vi "ExSubSetPixelResTifFileHeader.vi"(3 "error in (no error)":errorcluster, 4 "Camera Handle":u32, 5 "File Handle":u32) -> (0 "error out":errorcluster, 1 "Camera Handle":u32, 2 "File Handle":u32)   [LabVIEW 2010]
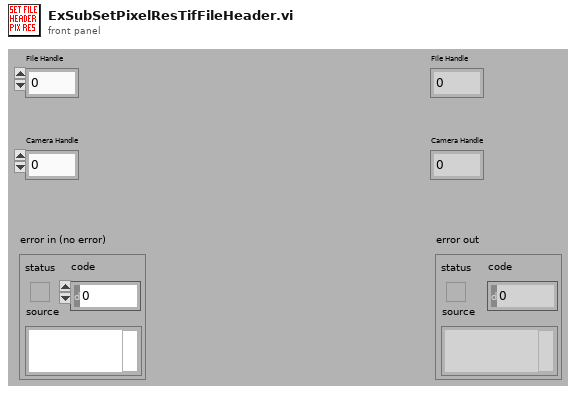
[diagram p1: front panel]
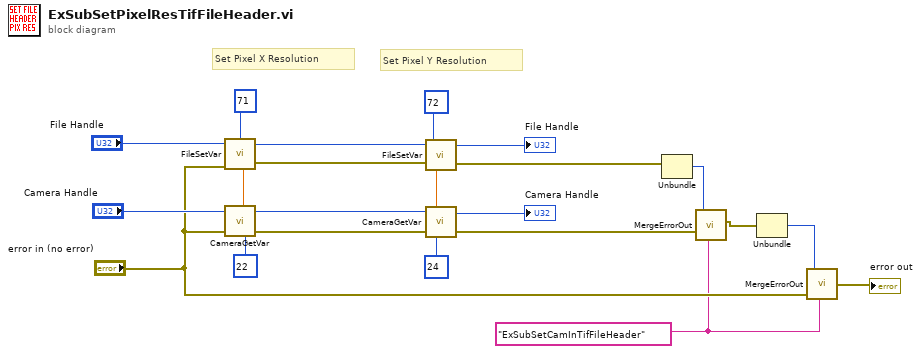
[diagram p0: block diagram]
diagram:
  w2 = "ExSubSetCamInTifFileHeader"
  # "Set Pixel Y Resolution"
  # "Set Pixel X Resolution"
  n1 = call <userlib>:"CameraGetVar.vi"("error in"="error in (no error)", "Parameter ID"=22, "Camera Handle"="Camera Handle") -> ("error out"=w15:errorcluster, "Value"=w20:dbl, "Camera Handle"=w16:u32)
  n2 = call <userlib>:"FileSetVar.vi"("error in"="error in (no error)", "Value"=w20, "Parameter ID"=71, "File Handle"="File Handle") -> ("error out"=w14:errorcluster, "File Handle"=w18:u32)
  n3 = call <userlib>:"CameraGetVar.vi"("error in"=w15, "Parameter ID"=24, "Camera Handle"=w16) -> ("error out"=w10:errorcluster, "Value"=w13:dbl, "Camera Handle"=→"Camera Handle":u32)
  n4 = call <userlib>:"FileSetVar.vi"("error in"=w14, "Value"=w13, "Parameter ID"=72, "File Handle"=w18) -> ("error out"=w11:errorcluster, "File Handle"=→"File Handle":u32)
  n5 = Unbundle(w11) -> ("code"=w12:i32)  [unwired: 2 out]
  n6 = call <userlib>:"MergeErrorOut.vi"("error in"=w10, "Fucntion Name"=w2, "ErrorCode"=w12) -> ("error out"=w4:errorcluster)
  n7 = Unbundle(w4) -> ("code"=w5:i32)  [unwired: 2 out]
  n8 = call <userlib>:"MergeErrorOut.vi"("error in"="error in (no error)", "Fucntion Name"=w2, "ErrorCode"=w5) -> ("error out"=→"error out":errorcluster)
